vi "Write next.vi"(10 "next":refnum<data-value>, 11 "Node in":refnum<class "Node.lvclass">) -> (3 "Node out":refnum<class "Node.lvclass">)   [LabVIEW 2023, in "d20.lvlib" / "Node.lvclass"]
uses:
  Node.lvclass
  INode/INode.lvclass
  Node.lvclass/Node.ctl
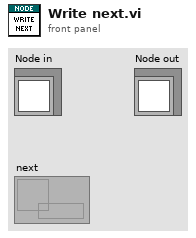
[diagram p1: front panel]
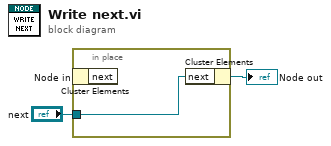
[diagram p0: block diagram]
diagram:
  n1 = in-place {
    in-place-border: "next" -> [w4]
    n2 = in-place-cluster #1("Node in") -> ()  [unwired: 1 out]
    n3 = in-place-cluster #1("next"=w4) -> (→"Node out":refnum<class "Node.lvclass">)
  }
